vi "auto mode.vi"(1 "What should the robot do?":T1(ring), 2 "What defense is in front of the robot?":T2(ring), 3 "Which defense position is the robot in front of?":enum16{"1", "2", "3", "4", "5", "Spy Box"}(ring)) -> ()   [LabVIEW 2015]
uses:
  <vilib>/Rock Robotics/Network Tables/NT Write Number.vi
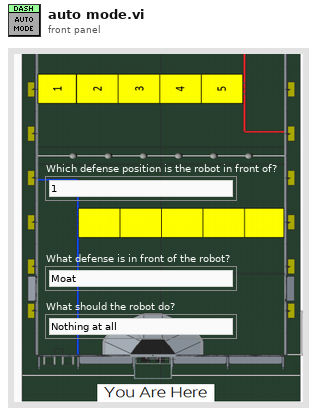
[diagram p1: front panel]
types:
  T1 = enum16{"Nothing at all", "Get to Defense", "Cross Defense", "Score High Goal", "Score Low Goal"}
  T2 = enum16{"Moat", "Ramparts", "Rock Wall", "Rough Terrain", "Something Else"}
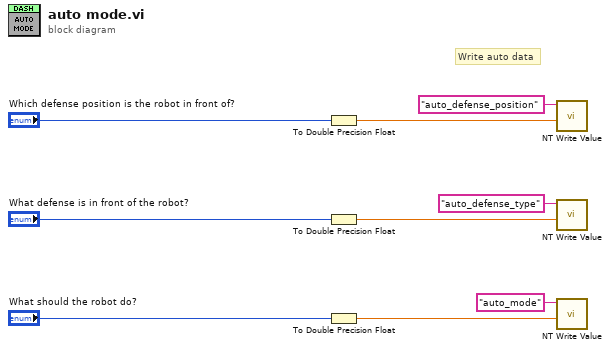
[diagram p0: block diagram]
diagram:
  # "Write auto data"
  n1 = To Double Precision Float(number="Which defense position is the robot in front of?") -> (double precision float=w8:dbl)
  n2 = To Double Precision Float(number="What defense is in front of the robot?") -> (double precision float=w7:dbl)
  n3 = To Double Precision Float(number="What should the robot do?") -> (double precision float=w2:dbl)
  n4 = call-poly <vilib>:"NT Write Value.vi"("Numeric"=w8, "Name"="auto_defense_position") -> ()  [unwired: 9 in, 1 out]
  n5 = call-poly <vilib>:"NT Write Value.vi"("Numeric"=w7, "Name"="auto_defense_type") -> ()  [unwired: 9 in, 1 out]
  n6 = call-poly <vilib>:"NT Write Value.vi"("Numeric"=w2, "Name"="auto_mode") -> ()  [unwired: 9 in, 1 out]
